vi "Event Handle Loop_Show Page.vi"(8 "error in (no error)":errorcluster, 10 "Page ID":string, 11 "QTab Class in":refnum<class "QTab Class.lvclass">) -> (0 "error out":errorcluster, 3 "QTab Class out":refnum<class "QTab Class.lvclass">)   [LabVIEW 2020, in "QTab.lvlib" / "QTab Class.lvclass"]
uses:
  QTab Class.lvclass
  QTab Class.lvclass/QTab Class.ctl
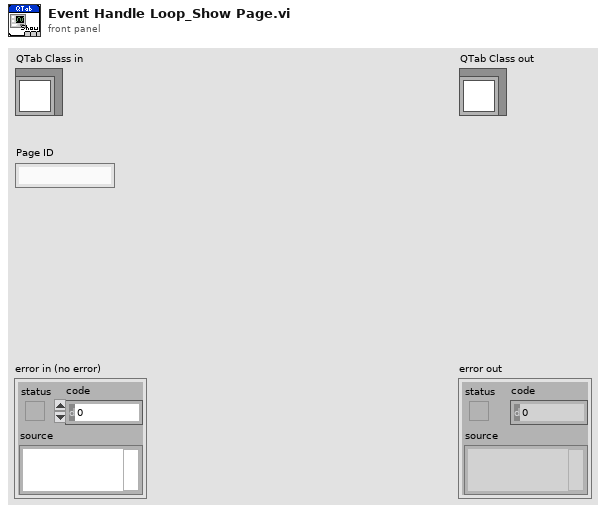
[diagram p1: front panel]
types:
  T1 = typedef "QTab.lvlib/QTab Class.lvclass/Pag Attribute.ctl" = cluster{"VI Refnum":refnum<vi>, "Page Name":string, "Closeable":bool, "Draggable":bool, "Pop-Out":bool}
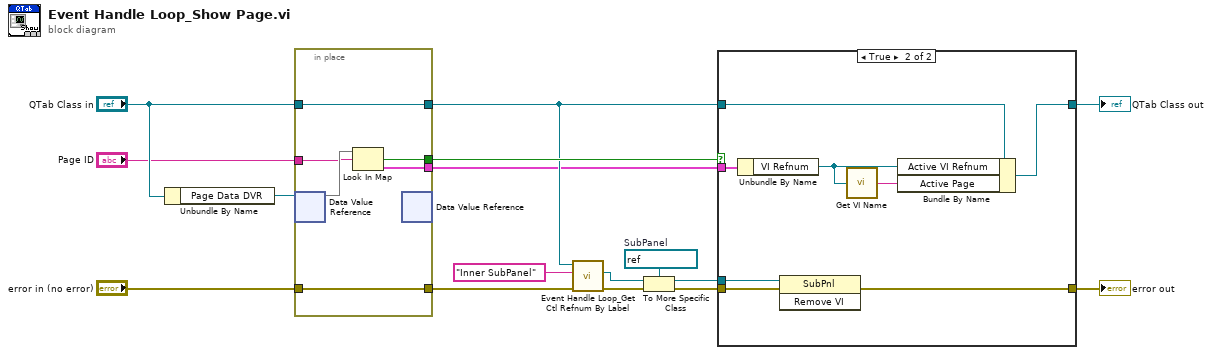
[diagram p0: block diagram]
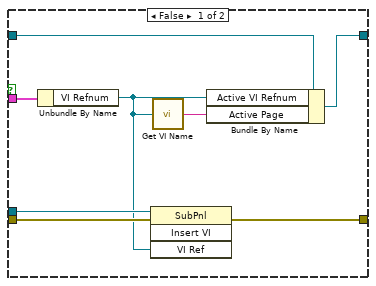
[diagram p2: hidden frame]
diagram:
  w6 = refnum<vi> refnum  # SubPanel
  n1 = Unbundle By Name("QTab Class in") -> ("Page Data DVR"=w15:refnum<data-value>)
  n2 = in-place {
    in-place-border: "QTab Class in" -> [w22]
    in-place-border: [w22] -> w8
    in-place-border: "error in (no error)" -> [w21]
    in-place-border: [w21] -> w9
    in-place-border: "Page ID" -> [w19]
    in-place-border: [w18] -> w10
    in-place-border: [w17] -> w7
    n3 = in-place-dvr #1(w15) -> (w20:map{string, T1})  [unwired: 1 out]
    n4 = Look In Map(map=w20, key=w19) -> (key not found?=w18:bool, value=w17:T1)  [unwired: 1 in]
    n5 = in-place-dvr #1() -> ()  [unwired: 1 in, 2 out]
  }
  n6 = call "Event Handle Loop_Get Ctl Refnum By Label.vi"("error in (no error)"=w9, "Label"="Inner SubPanel", "QTab Class in"=w8) -> ("error out"=w4:errorcluster, "Ctl Refnum"=w5:refnum<vi>)  [unwired: 6 in, 1 out]
  n7 = To More Specific Class(target class=w6, reference=w5, error in=w4) -> (specific class reference=w1:refnum<vi>, error out=w2:errorcluster)
  n8 = case shown="True" w10 {
    tunnel: [w30 w38] -> w16
    tunnel: w8 -> [w26 w34]
    tunnel: w2 -> [w28 w37]
    tunnel: [w25 w33] -> w11
    tunnel: w7 -> [w29 w35]
    tunnel: w1 -> [w27 w36]
    frame False {
      n9 = Unbundle By Name(w29) -> ("VI Refnum"=w23:refnum<vi>)
      n10 = invoke class="SubPnl" method="Insert VI"(reference=w27, error in=w28, "VI Ref"=w23) -> (error out=w30:errorcluster)  [unwired: 1 in, 3 out]
      n11 = call "Get VI Name.vi"("VI Refnum"=w23) -> ("VI Name"=w24:string)
      n12 = Bundle By Name(cluster=w26, "Active VI Refnum"=w23, "Active Page"=w24) -> (w25:refnum<class "QTab Class.lvclass">)
    }
    frame True {
      n13 = Unbundle By Name(w35) -> ("VI Refnum"=w31:refnum<vi>)
      n14 = invoke class="SubPnl" method="Remove VI"(reference=w36, error in=w37) -> (error out=w38:errorcluster)  [unwired: 1 in, 2 out]
      n15 = call "Get VI Name.vi"("VI Refnum"=w31) -> ("VI Name"=w32:string)
      n16 = Bundle By Name(cluster=w34, "Active VI Refnum"=w31, "Active Page"=w32) -> (w33:refnum<class "QTab Class.lvclass">)
    }
  }
  "error out" <- w16
  "QTab Class out" <- w11
